vi "place helicopter at height.vi"(10 "Image Arrays":T3, 11 "Arrays and Heights":T1={"Score Array"=[], "Lowest high score"=0.0, "Score"=0.0, "Ceiling"=0.0, "Floor"=0.0, "Ceiling Array"=[], "Floor array"=[], "Helicopter height"=0.0, "Helicopter array"=[], "Fuel"=300.0, "Fuel array"=[], "fuel counter"=0, "obstacle counter"=0, "Obstacle array"=[], "helicopter v_0"=0.0, "helicopter a_0"=0.0, "Obstacle height"=300.0}) -> (3 "Large image":u8[][](array[numeric]))   [LabVIEW 2017]
uses:
  controls/image arrays.ctl
  controls/arrays and heights.ctl
  controls/scores.ctl
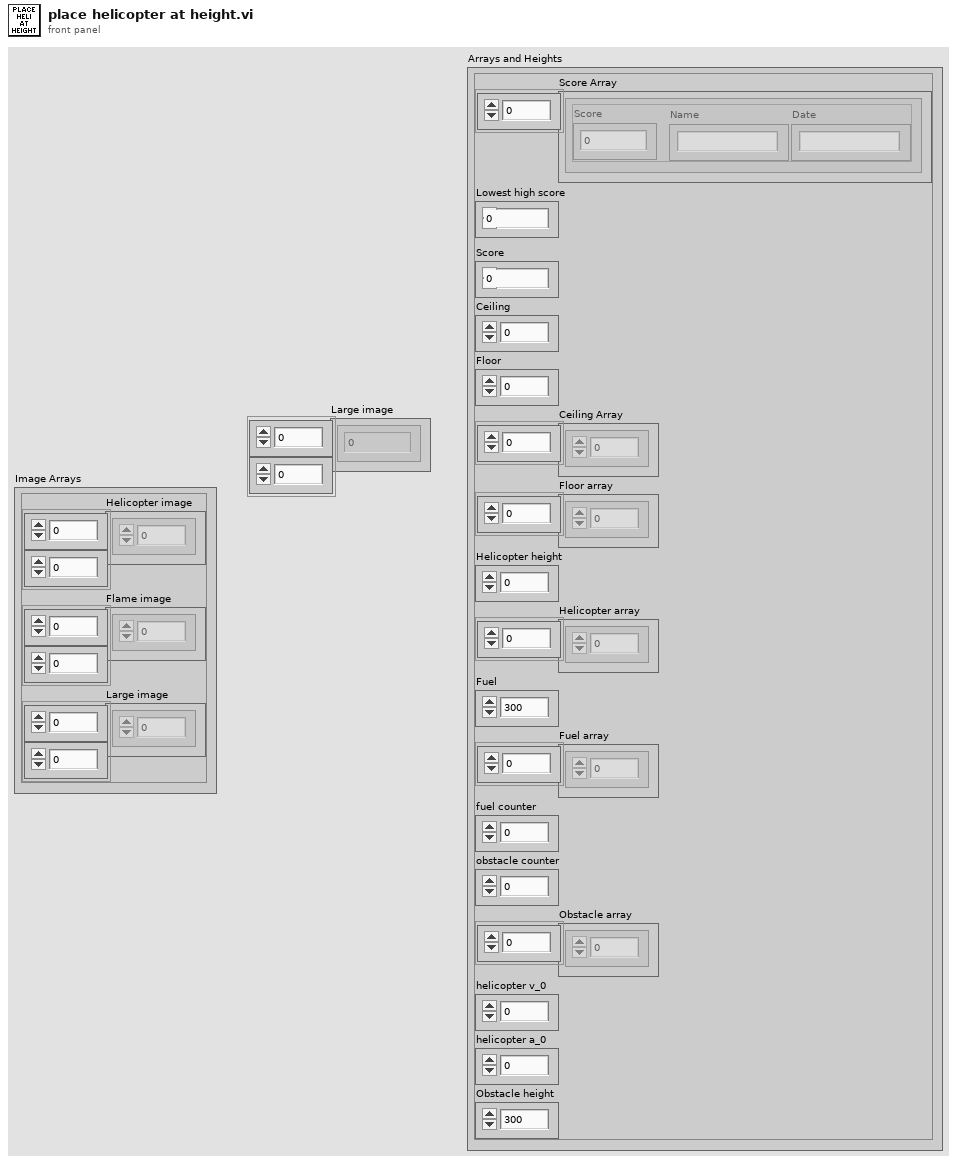
[diagram p1: front panel]
types:
  T1 = typedef "arrays and heights.ctl" = cluster{"Score Array":T2[], "Lowest high score":dbl, "Score":dbl, "Ceiling":dbl, "Floor":dbl, "Ceiling Array":dbl[], "Floor array":dbl[], "Helicopter height":dbl, "Helicopter array":dbl[], "Fuel":dbl, "Fuel array":dbl[], "fuel counter":i32, "obstacle counter":i32, "Obstacle array":dbl[], "helicopter v_0":dbl, "helicopter a_0":dbl, "Obstacle height":dbl}
  T2 = typedef "scores.ctl" = cluster{"Score":dbl, "Name":string, "Date":string}
  T3 = typedef "image arrays.ctl" = cluster{"Helicopter image":u8[][], "Flame image":u8[][], "Large image":u8[][]}
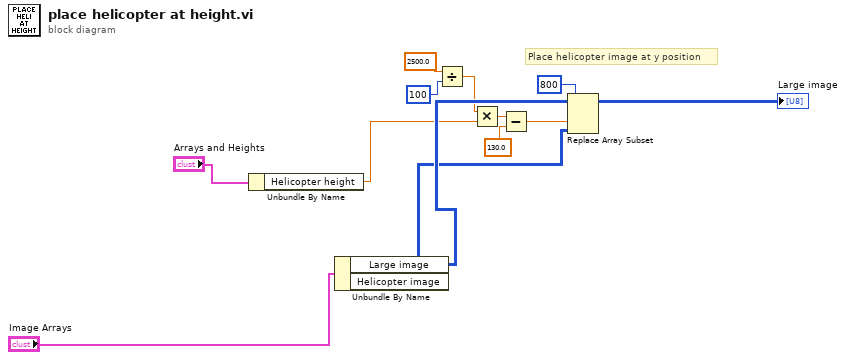
[diagram p0: block diagram]
diagram:
  # "Place helicopter image at y position"
  n1 = Unbundle By Name("Arrays and Heights") -> ("Helicopter height"=w1:dbl)
  n2 = Unbundle By Name("Image Arrays") -> ("Large image"=w13:u8[][], "Helicopter image"=w12:u8[][])
  n3 = Divide(x=2500.0, y=100) -> (x/y=w9:dbl)
  n4 = Multiply(x=w9, y=w1) -> (x*y=w5:dbl)
  n5 = Subtract(x=w5, y=130.0 ("y offset")) -> (x-y=w6:dbl)
  n6 = Replace Array Subset(array=w13, new element=w12, index (row)=800 ("disabled index (row)"), index (col)=w6) -> (→"Large image":u8[][])
